vi "Meres.vi"(6 "notifier":refnum<notifier>, 7 "queue":refnum<queue>, 8 "error in":errorcluster, 11 "Message Queues":T2) -> (0 "error":errorcluster)   [LabVIEW 2022 SP3]
uses:
  support/Message Queue/All Message Queues.ctl
  support/Message Queue/Message Cluster.ctl
  controls/Config.ctl
  controls/UI State.ctl
  <vilib>/Instr/_visa.llb/VISA Configure Serial Port (Instr).vi
  support/Message Queue/Message Queue.lvlib
  <vilib>/addons/Fuzzy Logic/NI_Fuzzy_Logic_API.lvlib
panel:
  in  "Settings":T1={"Hardware"={"VISA resource name"="COM3"}, "Logging"={"tdms file out"=refnum, "base path"=path ""}, "Set Temp"={"Numeric"=24.0}}
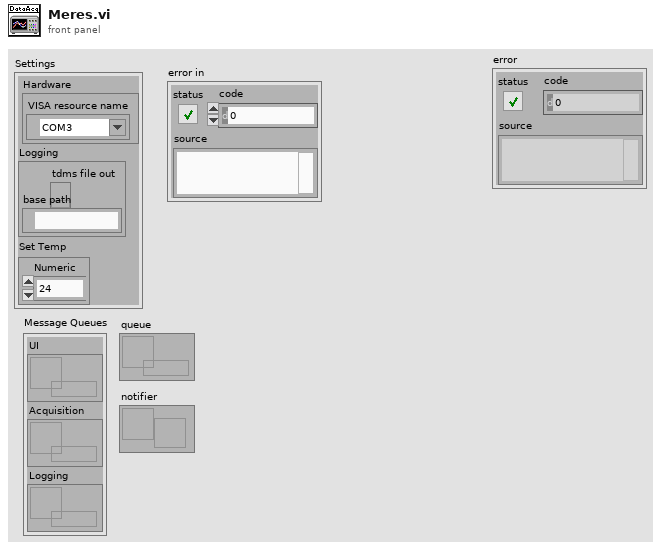
[diagram p1: front panel]
types:
  T1 = typedef "Config.ctl" = cluster{"Hardware":cluster{"VISA resource name":refnum<visa-resource-name>}, "Logging":cluster{"tdms file out":refnum<k34>, "base path":path}, "Set Temp":cluster{"Numeric":dbl}}
  T2 = typedef "Message Queue.lvlib/All Message Queues.ctl" = cluster{"UI":refnum<queue>, "Acquisition":refnum<queue>, "Logging":refnum<queue>}
  T3 = typedef "UI State.ctl" = enum16{"Idle", "Acquiring and logging", "Waiting for Exit", "Waiting for Stop"}
  T4 = typedef "NI_Fuzzy_Logic_API.lvlib/FL System.ctl" = cluster{"input variables":T5[], "output variables":T5[], "rules":T8[], "defuzzification method":T14, "description":string, "user MF interpolating polynomials":T15[]}
  T5 = typedef "NI_Fuzzy_Logic_API.lvlib/FL Variable.ctl" = cluster{"name":string, "range":dbl[], "MFs":T6[]}
  T6 = typedef "NI_Fuzzy_Logic_API.lvlib/FL Membership Function.ctl" = cluster{"name":string, "shape":T7, "points":dbl[], "color":u32, "user-defined shape index":i32}
  T7 = typedef "NI_Fuzzy_Logic_API.lvlib/FL Membership Function Shape.ctl" = u16
  T8 = typedef "NI_Fuzzy_Logic_API.lvlib/FL Rule.ctl" = cluster{"antecedents":T9[], "antecedent connective":T11, "consequents":T12[], "consequent implication":T13, "degree of support":dbl}
  T9 = typedef "NI_Fuzzy_Logic_API.lvlib/FL Antecedent.ctl" = cluster{"Var Index":i32, "MF Index":i32, "Cond":T10}
  T10 = typedef "NI_Fuzzy_Logic_API.lvlib/FL Modifier.ctl" = u16
  T11 = typedef "NI_Fuzzy_Logic_API.lvlib/FL Antecedent Connective.ctl" = u16
  T12 = typedef "NI_Fuzzy_Logic_API.lvlib/FL Consequent.ctl" = cluster{"Var Index":i32, "MF Index":i32, "Cond":T10}
  T13 = typedef "NI_Fuzzy_Logic_API.lvlib/FL Consequent Implication.ctl" = u16
  T14 = typedef "NI_Fuzzy_Logic_API.lvlib/FL Defuzzification.ctl" = u16
  T15 = typedef "NI_Fuzzy_Logic_API.lvlib/FL Interpolating polynomials.ctl" = cluster{"X":dbl[], "Y":dbl[], "Y(x) coeff":dbl[][], "X(y) coeff":dbl[][], "Area(y) coeff":dbl[][], "coa_x(y) coeff":dbl[][]}
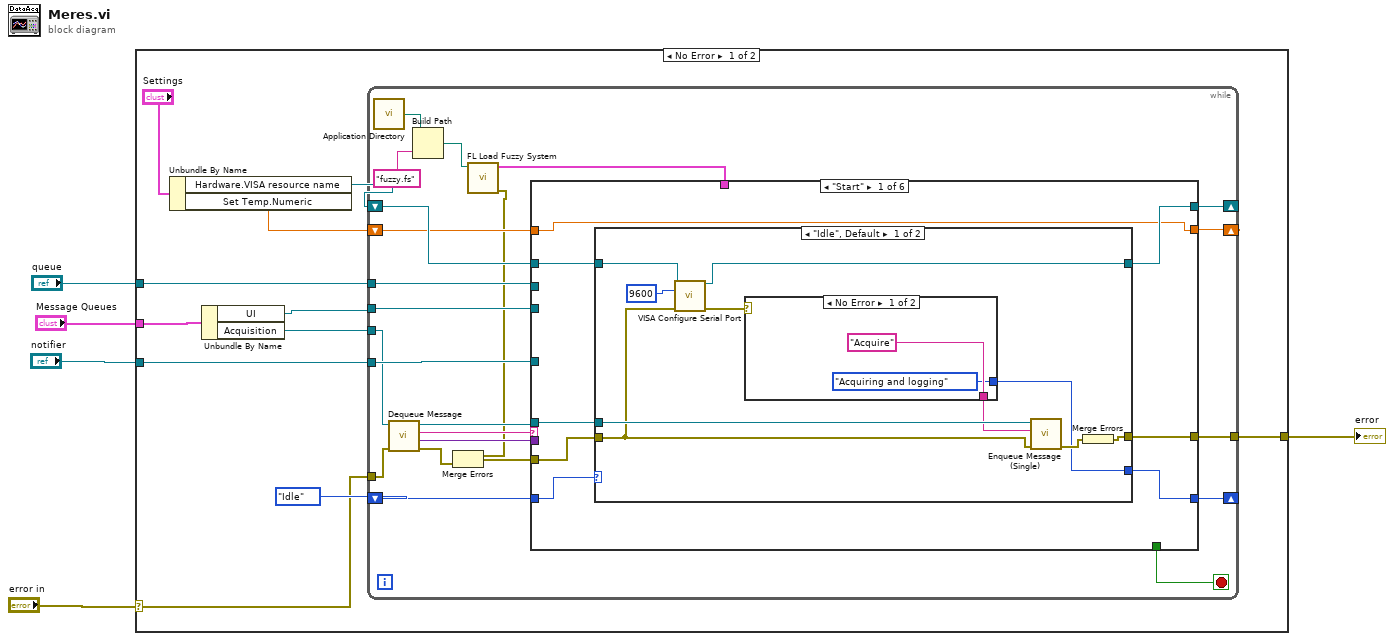
[diagram p0: block diagram]
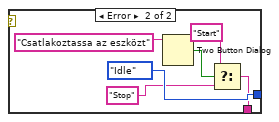
[diagram p2: hidden frame]
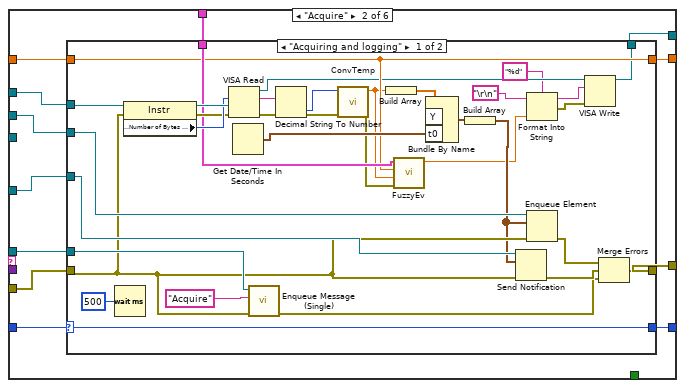
[diagram p4: hidden frame]
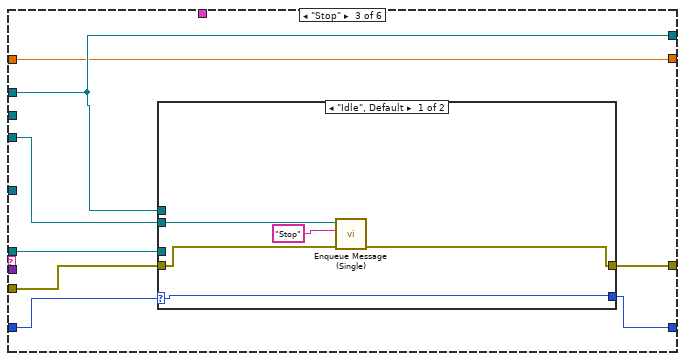
[diagram p6: hidden frame]
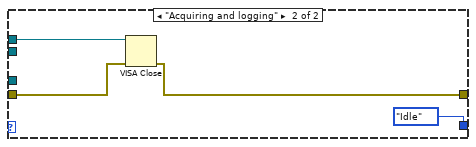
[diagram p7: hidden frame]
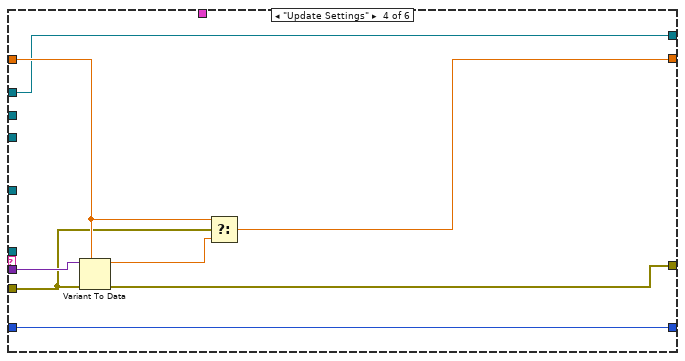
[diagram p8: hidden frame]
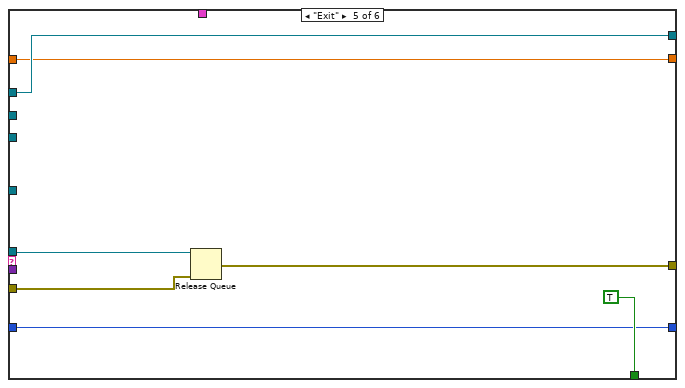
[diagram p9: hidden frame]
diagram:
  n1 = case shown="No Error" "error in" {
    selector: "error in" -> [w9 w154]
    tunnel: "notifier" -> [w15 _]
    tunnel: "Message Queues" -> [w14 _]
    tunnel: "queue" -> [w13 _]
    tunnel: [w10 w154] -> w1
    frame No Error {
      n2 = Unbundle By Name("Settings") -> ("Hardware.VISA resource name"=w12:refnum<visa-resource-name>, "Set Temp.Numeric"=w6:dbl)
      n3 = Unbundle By Name(w14) -> ("UI"=w11:refnum<queue>, "Acquisition"=w8:refnum<queue>)
      n4 = while {
        shift-right: [w38] -> _
        shift-left: UI_State."Idle" ("Enum") -> [w39]
        tunnel: w15 -> [w33]
        tunnel: w13 -> [w34]
        shift-right: [w36] -> _
        shift-left: w12 -> [w37]
        tunnel: w11 -> [w32]
        tunnel: [w35] -> w10
        tunnel: w9 -> [w30]
        tunnel: w8 -> [w29]
        shift-right: [w24] -> _
        shift-left: w6 -> [w25]
        stop <- w31 stop-if-true
        n5 = call <vilib>:"Application Directory.vi"() -> ("Application Directory"=w18:path)
        n6 = call "Dequeue Message.vi"("error in (no error)"=w30, "Message Queue"=w29) -> ("error out"=w20:errorcluster, "Message Data"=w28:variant, "Message"=w27:string, "dup Message Queue"=w26:refnum<queue>)  [unwired: 6 in]
        n7 = Build Path(base path=w18, name or relative path="fuzzy.fs") -> (appended path=w19:path)
        n8 = call <vilib>:"FL Load Fuzzy System.vi"("file path"=w19) -> ("error out"=w21:errorcluster, "fuzzy system out"=w23:T4)  [unwired: 9 in]
        n9 = Merge Errors(w21, w20) -> (w22:errorcluster)
        n10 = case shown="\"Start\"" w27 {
          tunnel: w39 -> [w47 w80 w125 w140 w144 w152]
          tunnel: [w42 w79 w122 w140 w144 w152] -> w38
          tunnel: w28 -> [_ _ _ w142 _ _]
          tunnel: w22 -> [w45 w76 w124 w136 w146 w150]
          tunnel: w37 -> [w46 w78 w121 w137 w149 w153]
          tunnel: [w44 w77 w121 w137 w149 w153] -> w36
          tunnel: w26 -> [w43 w74 w120 _ w147 _]
          tunnel: [w41 w75 w123 w135 w145 w150] -> w35
          tunnel: w34 -> [_ w73 _ _ _ _]
          tunnel: w33 -> [_ w72 _ _ _ _]
          tunnel: w32 -> [_ _ w119 _ _ _]
          tunnel: [_ _ _ _ TRUE _] -> w31
          tunnel: w25 -> [w40 w71 w118 w139 w143 w151]
          tunnel: [w40 w70 w118 w138 w143 w151] -> w24
          tunnel: w23 -> [_ w69 _ _ _ _]
          frame "Start" {
            n11 = case shown="\"Idle\", Default" w47 {
              selector: w47 -> [_ w67]
              tunnel: w46 -> [w49 w66]
              tunnel: w45 -> [w53 w68]
              tunnel: [w48 w66] -> w44
              tunnel: w43 -> [w56 _]
              tunnel: [w51 w67] -> w42
              tunnel: [w54 w68] -> w41
              frame "Idle", Default {
                n12 = call-poly "VISA Configure Serial Port"("VISA resource name"=w49, "baud rate (9600)"=u32 9600, "error in (no error)"=w53) -> ("VISA resource name out"=w48:refnum<visa-resource-name>, "error out"=w50:errorcluster)  [unwired: 11 in]
                n13 = case shown="No Error" w50 {
                  tunnel: ["Acquire" ("Message") w61] -> w52
                  tunnel: [UI_State."Acquiring and logging" ("Enum") UI_State."Idle" ("Enum")] -> w51
                  frame No Error {
                  }
                  frame Error {
                    n14 = Two Button Dialog(message="Csatlakoztassa az eszközt") -> (T button?=w63:bool)  [unwired: 2 in]
                    n15 = Select(t="Start" ("Message"), s=w63, f="Stop" ("Message")) -> (s? t:f=w61:string)
                  }
                }
                n16 = call "Enqueue Message (Single).vi"("error in (no error)"=w53, "Message"=w52, "Message Queue"=w56) -> ("error out"=w55:errorcluster)  [unwired: 7 in, 1 out]
                n17 = Merge Errors(w55) -> (w54:errorcluster)
              }
              frame "Acquiring and logging" {
              }
            }
          }
          frame "Acquire" {
            n18 = case shown="\"Acquiring and logging\"" w80 {
              selector: w80 -> [w97 w117]
              tunnel: [w97 w117] -> w79
              tunnel: w78 -> [w98 w116]
              tunnel: [w84 w116] -> w77
              tunnel: [w88 w115] -> w75
              tunnel: w76 -> [w104 w115]
              tunnel: w74 -> [w113 _]
              tunnel: w73 -> [w111 _]
              tunnel: w72 -> [w110 _]
              tunnel: [w94 w114] -> w70
              tunnel: w71 -> [w94 w114]
              tunnel: w69 -> [w95 _]
              frame "Acquiring and logging" {
                n19 = Wait (ms)(milliseconds to wait=u32 500) -> ()  [unwired: 1 out]
                n20 = property class="Instr"(reference=w98, error in=w104) -> (reference out=w109:refnum<visa-resource-name>, error out=w103:errorcluster, "Serial Settings:Number of Bytes at Serial Port"=w108:u32)
                n21 = VISA Read(VISA resource name=w109, byte count=w108, error in (no error)=w103) -> (VISA resource name out=w87:refnum<visa-resource-name>, read buffer=w105:string, error out=w101:errorcluster)  [unwired: 1 out]
                n22 = Get Date/Time In Seconds() -> (seconds since 1Jan1904=w107:timestamp)
                n23 = call "Enqueue Message (Single).vi"("error in (no error)"=w104, "Message"="Acquire", "Message Queue"=w113) -> ("error out"=w89:errorcluster)  [unwired: 7 in, 1 out]
                n24 = Decimal String To Number(string=w105) -> (number=w102:i32)  [unwired: 2 in, 1 out]
                n25 = call "ConvTemp.vi"("error constant"=w101, "DataIn"=w102) -> ("error constant 2"=w92:errorcluster, "Temperature"=w93:dbl)  [unwired: 8 in]
                n26 = Build Array(w93) -> (w100:dbl[])
                n27 = call "FuzzyEv.vi"("error in (no error)"=w92, "Temp"=w93, "SetTemp"=w94, "fuzzy system in"=w95) -> ("output value"=w85:dbl)  [unwired: 6 in, 1 out]
                n28 = Bundle By Name("Y"=w100, "t0"=w107) -> (w106:waveform(dbl))  [unwired: 1 in]
                n29 = Build Array(w106) -> (w96:waveform(dbl)[])
                n30 = Send Notification(notification=w96, notifier=w110, error in (no error)=w104) -> (error out=w90:errorcluster)  [unwired: 1 out]
                n31 = Format Into String(format string="%d", initial string="\r\n", w85) -> (resulting string=w81:string, error out=w86:errorcluster)  [unwired: 1 in]
                n32 = Enqueue Element(queue=w111, element=w96, error in (no error)=w104) -> (error out=w91:errorcluster)  [unwired: 1 in, 2 out]
                n33 = VISA Write(VISA resource name=w87, write buffer=w81, error in (no error)=w86) -> (VISA resource name out=w84:refnum<visa-resource-name>)  [unwired: 2 out]
                n34 = Merge Errors(w91, w90, w89) -> (w88:errorcluster)
              }
              frame "Idle", Default {
              }
            }
          }
          frame "Stop" {
            n35 = case shown="\"Idle\", Default" w125 {
              selector: w125 -> [w130 _]
              tunnel: w124 -> [w127 w134]
              tunnel: [w126 w131] -> w123
              tunnel: [w130 UI_State."Idle" ("Enum")] -> w122
              tunnel: w121 -> [_ w132]
              tunnel: w120 -> [_ _]
              tunnel: w119 -> [w129 _]
              frame "Idle", Default {
                n36 = call "Enqueue Message (Single).vi"("error in (no error)"=w127, "Message"="Stop", "Message Queue"=w129) -> ("error out"=w126:errorcluster)  [unwired: 7 in, 1 out]
              }
              frame "Acquiring and logging" {
                n37 = VISA Close(VISA resource name=w132, error in (no error)=w134) -> (error out=w131:errorcluster)
              }
            }
          }
          frame "Update Settings" {
            n38 = Variant To Data(error in=w136, type=w139, Variant=w142) -> (data=w141:dbl, error out=w135:errorcluster)
            n39 = Select(t=w139, s=w136, f=w141) -> (s? t:f=w138:dbl)
          }
          frame "Exit" {
            n40 = Release Queue(queue=w147, error in (no error)=w146) -> (error out=w145:errorcluster)  [unwired: 1 in, 2 out]
          }
          frame Default {
          }
        }
      }
    }
    frame Error {
    }
  }
  "error" <- w1
